vi "RP read signal channel.vi"(7 "Pipeline delay":dbl=28.0, 8 "Error In":errorcluster, 9 "Channel name":string, 10 "group name in":string, 11 "File":path) -> (0 "Error Out":errorcluster, 1 "Phase":dbl, 2 "Frequency":dbl format="%_19p", 3 "Data out":waveform(dbl), 4 "Phase word":u32, 5 "Frequency word":u32, 6 "File out":path)   [LabVIEW 2016]
panel:
  out "t0":dbl format="%#_6p"
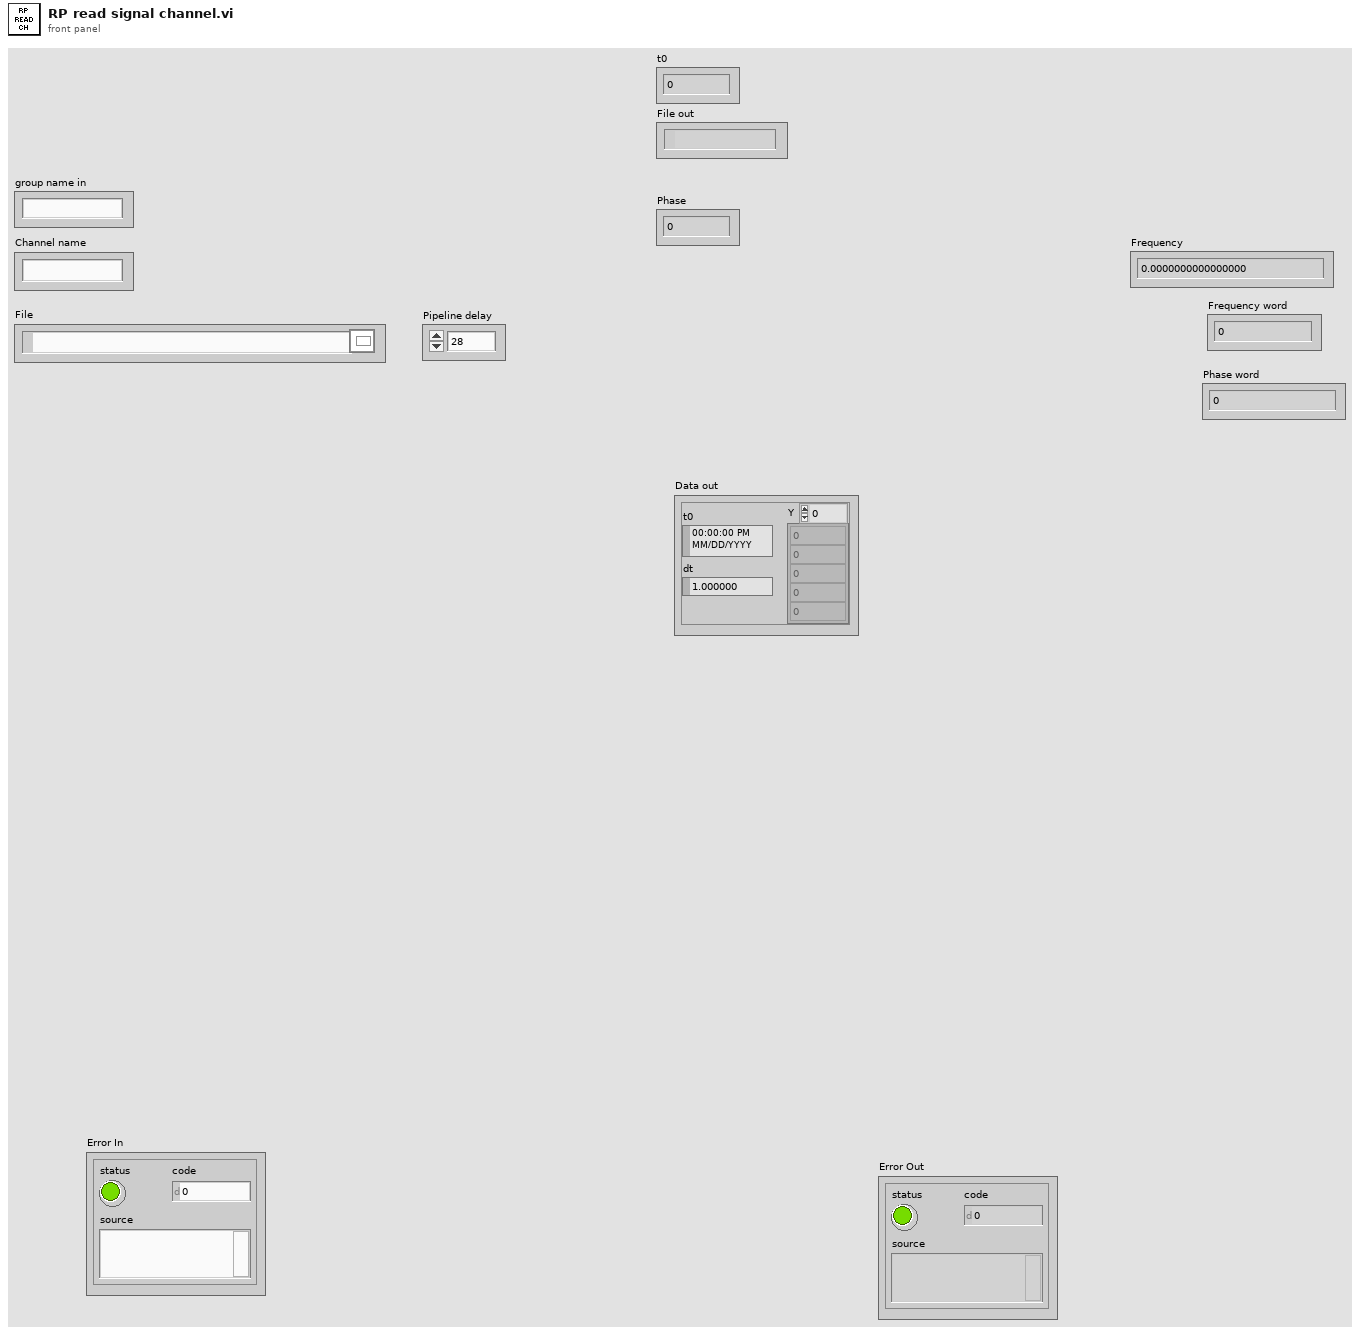
[diagram p1: front panel]
types:
  T1 = enum16{"open", "open or create", "create or replace", "create", "open (read-only)"}
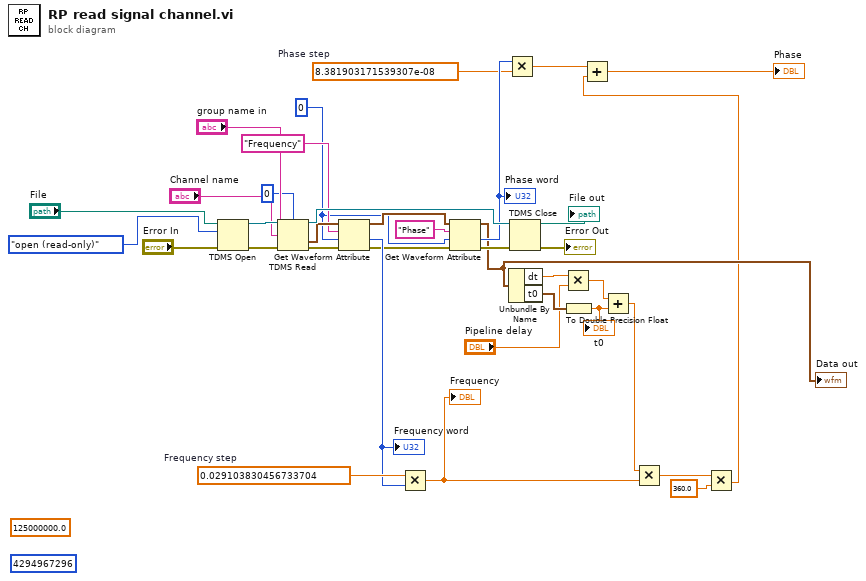
[diagram p0: block diagram]
diagram:
  w10 = u32 0 ("index")
  w26 = 8.381903171539307e-08  # Phase step
  w29 = 0.029103830456733704  # Frequency step
  (unwired) u64 4294967296
  (unwired) 125000000.0
  n1 = TDMS Open(8:"Error In", 10:T1."open (read-only)" ("operation (0:open)"), 11:"File") -> (0:w33:errorcluster, 3:w32:refnum<k34>)  [unwired: 4 in]
  n2 = TDMS Read(0:w32, 2:i64 0 ("count (-1: all)"), 5:"group name in", 7:"Channel name", 11:w33) -> (4:w31:refnum<k34>, 10:w16:waveform(dbl), 15:w14:errorcluster)  [unwired: 3 in, 3 out]
  n3 = Get Waveform Attribute(4:w14, 5:w10, 6:"Frequency" ("name"), 7:w16) -> (0:w12:errorcluster, 1:w28:u32, 3:w13:waveform(dbl))  [unwired: 1 out]
  "Frequency word" <- w28
  n4 = Multiply(x=w29, y=w28) -> (x*y=w25:dbl)
  "Frequency" <- w25
  n5 = Get Waveform Attribute(4:w12, 5:w10, 6:"Phase" ("name"), 7:w13) -> (0:w30:errorcluster, 1:w27:u32, 3:w7:waveform(dbl))  [unwired: 1 out]
  "Phase word" <- w27
  "Data out" <- w7
  n6 = Multiply(x=w27, y=w26) -> (x*y=w4:dbl)
  n7 = Unbundle By Name(w7) -> ("dt"=w19:dbl, "t0"=w21:timestamp)
  n8 = TDMS Close(8:w30, 11:w31) -> (0:→"Error Out":errorcluster, 3:→"File out":path)
  n9 = Multiply(x=w19, y="Pipeline delay") -> (x*y=w17:dbl)
  n10 = To Double Precision Float(number=w21) -> (double precision float=w24:dbl)
  "t0" <- w24
  n11 = Add(x=w17, y=w24) -> (x+y=w18:dbl)
  n12 = Multiply(x=w18, y=w25) -> (x*y=w23:dbl)
  n13 = Multiply(x=w23, y=360.0) -> (x*y=w5:dbl)
  n14 = Add(x=w4, y=w5) -> (x+y=→"Phase":dbl)
